vi "Read App Config.vi"(11 "App Config Path":path) -> (2 "Cal Files Path":path, 3 "Registered Systems":T1[](array[typedef]))   [LabVIEW 2019]
uses:
  Type Defs/Registered System.ctl
  Type Defs/System Type.ctl
  <vilib>/Utility/config.llb/Read Key (Path).vi
  <vilib>/Utility/config.llb/Read Key (String).vi
  <vilib>/Utility/config.llb/Write Key (Path).vi
  <vilib>/Utility/config.llb/NI_LVConfig.lvlib
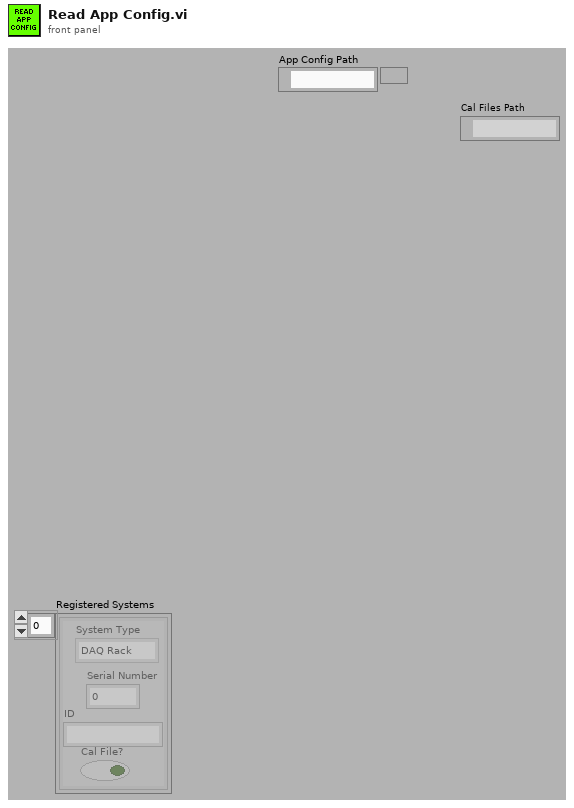
[diagram p1: front panel]
types:
  T1 = typedef "Registered System.ctl" = cluster{"System Type":T2, "Serial Number":u32, "ID":string, "Cal File?":bool}
  T2 = typedef "System Type.ctl" = enum16{"DAQ Rack", "DAQ Cart", "RIO", "unknown", "open"}
  T3 = typedef "NI_LVConfig.lvlib/Config Data RefNum.ctl" = refnum<k1>
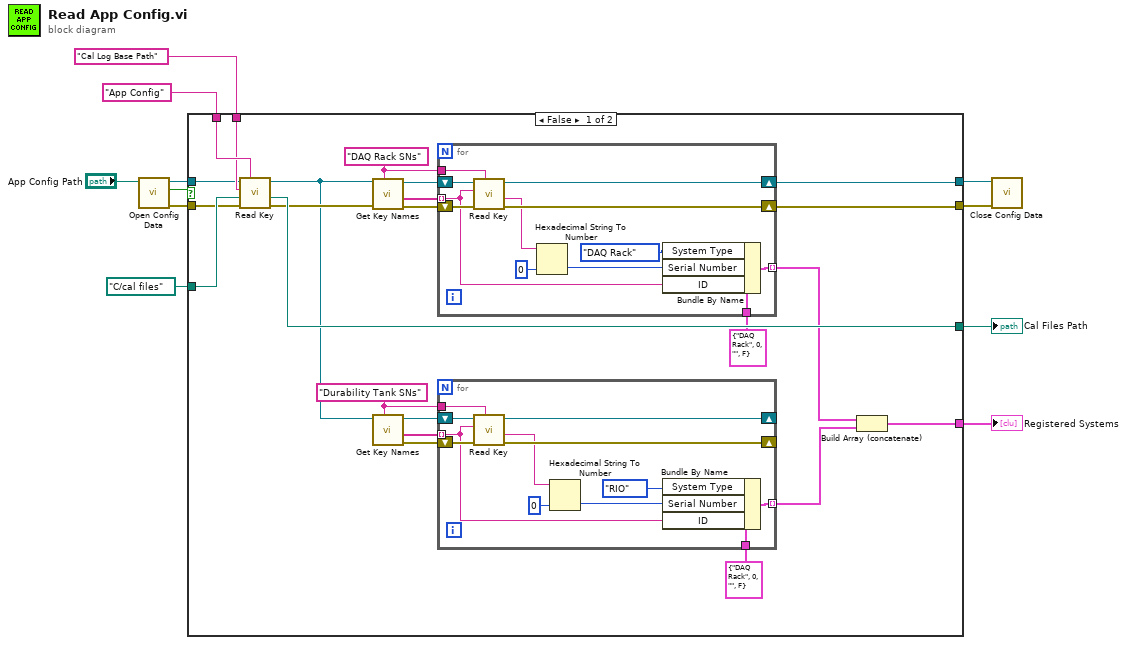
[diagram p0: block diagram]
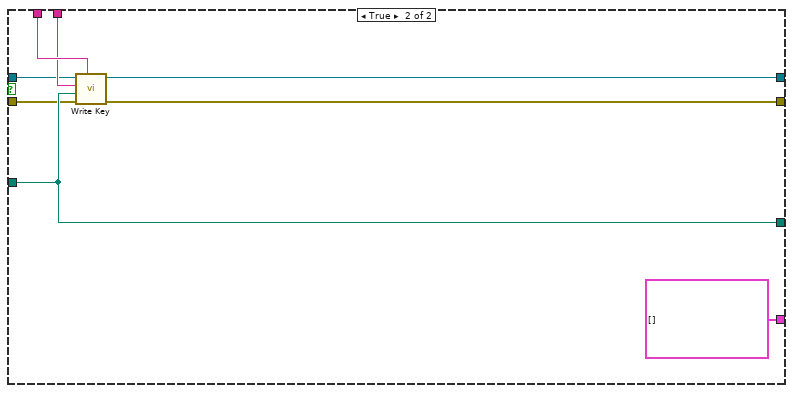
[diagram p2: hidden frame]
diagram:
  n1 = call <vilib>:"Open Config Data.vi"("configuration file path"="App Config Path") -> ("error out"=w5:errorcluster, "file created?"=w10:bool, "refnum"=w6:T3)  [unwired: 8 in]
  n2 = case shown="False" w10 {
    tunnel: w5 -> [w30 w62]
    tunnel: w6 -> [w31 w63]
    tunnel: "App Config" ("section") -> [w33 w65]
    tunnel: [w14 w61] -> w8
    tunnel: [w15 w60] -> w9
    tunnel: path "C:/cal files" ("default value") -> [w34 w66]
    tunnel: [w29 w66] -> w3
    tunnel: "Cal Log Base Path" ("section") -> [w32 w64]
    tunnel: [w13 T1[] []] -> w1
    frame False {
      w26 = "Durability Tank SNs" ("section")
      w17 = "DAQ Rack SNs" ("section")
      n3 = call-poly <vilib>:"Read Key.vi"("section"=w33, "error in (no error)"=w30, "default value"=w34, "key"=w32, "refnum"=w31) -> ("error out"=w16:errorcluster, "value"=w29:path, "refnum out"=w12:T3)  [unwired: 3 in, 1 out]
      n4 = call <vilib>:"Get Key Names.vi"("section"=w17, "error in (no error)"=w16, "refnum"=w12) -> ("error out"=w19:errorcluster, "key names"=w18:string[], "refnum out"=w20:T3)  [unwired: 5 in, 1 out]
      n5 = call <vilib>:"Get Key Names.vi"("section"=w26, "refnum"=w12) -> ("error out"=w24:errorcluster, "key names"=w25:string[], "refnum out"=w23:T3)  [unwired: 6 in, 1 out]
      n6 = for {
        tunnel: w17 -> [w58]
        tunnel: w18 -> [w49] mode=indexing
        shift-right: [w56] -> w14
        shift-left: w19 -> [w57]
        shift-right: [w54] -> w15
        shift-left: w20 -> [w55]
        tunnel: T1 {"System Type"=enum."DAQ Rack", "Serial Number"=0, "ID"="", "Cal File?"=FALSE} ("Cluster") -> [w51]
        tunnel: [w48] -> w27 mode=indexing
        n7 = call-poly <vilib>:"Read Key.vi"("section"=w58, "error in (no error)"=w57, "key"=w49, "refnum"=w55) -> ("error out"=w56:errorcluster, "value"=w53:string, "refnum out"=w54:T3)  [unwired: 4 in, 1 out]
        n8 = Hexadecimal String To Number(string=w53, default (0uL)=u32 0 ("default (0 U32)")) -> (number=w50:u32)  [unwired: 1 in, 1 out]
        n9 = Bundle By Name(cluster=w51, "System Type"=System_Type."DAQ Rack", "Serial Number"=w50, "ID"=w49) -> (w48:T1)
      }
      n10 = for {
        tunnel: w26 -> [w46]
        tunnel: w25 -> [w37] mode=indexing
        shift-right: [w44] -> _
        shift-left: w24 -> [w45]
        shift-right: [w42] -> _
        shift-left: w23 -> [w43]
        tunnel: T1 {"System Type"=enum."DAQ Rack", "Serial Number"=0, "ID"="", "Cal File?"=FALSE} ("Cluster") -> [w39]
        tunnel: [w36] -> w28 mode=indexing
        n11 = call-poly <vilib>:"Read Key.vi"("section"=w46, "error in (no error)"=w45, "key"=w37, "refnum"=w43) -> ("error out"=w44:errorcluster, "value"=w41:string, "refnum out"=w42:T3)  [unwired: 4 in, 1 out]
        n12 = Hexadecimal String To Number(string=w41, default (0uL)=u32 0 ("default (0 U32)")) -> (number=w38:u32)  [unwired: 1 in, 1 out]
        n13 = Bundle By Name(cluster=w39, "System Type"=System_Type."RIO", "Serial Number"=w38, "ID"=w37) -> (w36:T1)
      }
      n14 = Build Array (concatenate)(w27, w28) -> (w13:T1[])
    }
    frame True {
      n15 = call-poly <vilib>:"Write Key.vi"("section"=w65, "error in (no error)"=w62, "value"=w66, "key"=w64, "refnum"=w63) -> ("error out"=w61:errorcluster, "refnum out"=w60:T3)  [unwired: 4 in, 1 out]
    }
  }
  "Cal Files Path" <- w3
  "Registered Systems" <- w1
  n16 = call <vilib>:"Close Config Data.vi"("error in (no error)"=w8, "refnum"=w9) -> ()  [unwired: 8 in, 2 out]
